vi "I2C Read Data.vi"(5 "Address":T1 format="%02x", 6 "NoStop (F)":bool, 7 "I2C #":T2=-1, 8 "error in (no error)":errorcluster, 9 "Len":u8, 11 "VisaComms in":refnum<class "VisaComms.lvclass">) -> (0 "error out":errorcluster, 1 "Data":string, 3 "VisaComms out":refnum<class "VisaComms.lvclass">)   [LabVIEW 2020, in "CTI.lvlib" / "VisaComms.lvclass"]
uses:
  VisaComms.lvclass
  VisaComms.lvclass/VisaComms.ctl
  I2C Number.ctl
  CTI.lvlib
  I2C Address.ctl
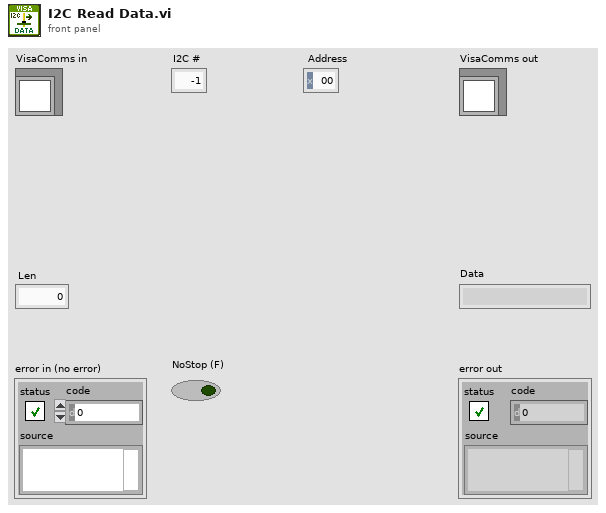
[diagram p1: front panel]
types:
  T1 = typedef "CTI.lvlib/I2C Address.ctl" = u8
  T2 = typedef "CTI.lvlib/I2C Number.ctl" = i8
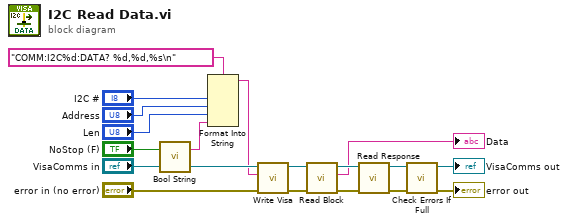
[diagram p0: block diagram]
diagram:
  n1 = call "Bool String.vi"("Bool"="NoStop (F)") -> ("String"=w12:string)  [unwired: 6 in]
  n2 = Format Into String(format string="COMM:I2C%d:DATA? %d,%d,%s\n", "I2C #", "Address", "Len", w12) -> (resulting string=w10:string)  [unwired: 2 in, 1 out]
  n3 = call "Write Visa.vi"("error in (no error)"="error in (no error)", "write buffer"=w10, "VisaComms in"="VisaComms in") -> ("error out"=w9:errorcluster, "VisaComms out"=w7:refnum<class "VisaComms.lvclass">)  [unwired: 6 in, 1 out]
  n4 = call "Read Block.vi"("error in (no error)"=w9, "VisaComms in"=w7) -> ("error out"=w8:errorcluster, "Block"=→"Data":string, "VisaComms out"=w5:refnum<class "VisaComms.lvclass">)  [unwired: 7 in]
  n5 = call "Read Response.vi"("error in (no error)"=w8, "VisaComms in"=w5) -> ("error out"=w6:errorcluster, "VisaComms out"=w2:refnum<class "VisaComms.lvclass">)  [unwired: 7 in, 1 out]
  n6 = call "Check Errors If Full.vi"("error in (no error)"=w6, "VisaComms in"=w2) -> ("error out"=→"error out":errorcluster, "VisaComms out"=→"VisaComms out":refnum<class "VisaComms.lvclass">)  [unwired: 8 in]
